vi "Remove Service.vi"(8 "error in (no error)":errorcluster, 10 "Class Name":string, 11 "Server in":refnum<class "Server.lvclass">) -> (0 "error out":errorcluster, 3 "Server out":refnum<class "Server.lvclass">)   [LabVIEW 2024, in "Ramses Framework.lvlib" / "Server.lvclass"]
uses:
  Server.lvclass
  Server.lvclass/Server.ctl
  Service/Service.lvclass
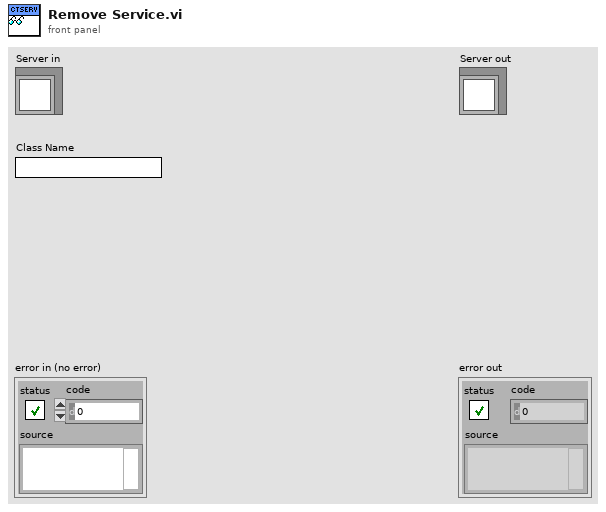
[diagram p1: front panel]
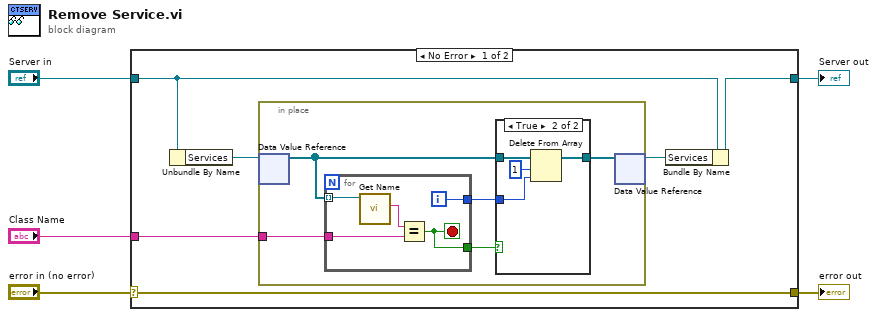
[diagram p0: block diagram]
diagram:
  n1 = case shown="No Error" "error in (no error)" {
    selector: "error in (no error)" -> [w11 w28]
    tunnel: [w11 w28] -> w4
    tunnel: "Server in" -> [w9 w27]
    tunnel: "Class Name" -> [w10 _]
    tunnel: [w8 w27] -> w1
    frame No Error {
      n2 = Unbundle By Name(w9) -> ("Services"=w7:refnum<data-value>)
      n3 = in-place {
        in-place-border: w10 -> [w16]
        n4 = in-place-dvr #1(w7) -> (w13:refnum<class "Service.lvclass">[])  [unwired: 1 out]
        n5 = for {
          tunnel: w13 -> [w26] mode=indexing
          tunnel: w16 -> [w24]
          tunnel: [w23] -> w15
          tunnel: [w22] -> w14
          i -> [w22]
          stop <- w23 stop-if-true
          n6 = call "Get Name.vi"("Service in"=w26) -> ("Name"=w25:string)  [unwired: 8 in, 2 out]
          n7 = Equal?(x=w25, y=w24) -> (x = y?=w23:bool)
        }
        n8 = case shown="True" w15 {
          tunnel: w14 -> [_ w20]
          tunnel: w13 -> [w17 w21]
          tunnel: [w17 w18] -> w12
          frame False {
          }
          frame True {
            n9 = Delete From Array(array=w21, length=1, index=w20) -> (array with subset deleted=w18:refnum<class "Service.lvclass">[])  [unwired: 1 out]
          }
        }
        n10 = in-place-dvr #1(w12) -> (w6:refnum<data-value>)  [unwired: 1 out]
      }
      n11 = Bundle By Name(cluster=w9, "Services"=w6) -> (w8:refnum<class "Server.lvclass">)
    }
    frame Error {
    }
  }
  "error out" <- w4
  "Server out" <- w1
